vi "CylSetSeq.vi"(8 "error in (no error)":errorcluster, 9 "Delay Time":dbl[unit] format="%.3f", 10 "SEQ in":refnum<class "Sequence.lvclass">, 11 "Cycle in":refnum<class "Cycle.lvclass">) -> (0 "error out":errorcluster, 3 "Cycle out":refnum<class "Cycle.lvclass">)   [LabVIEW 2012, in "Cycle.lvclass"]
uses:
  Cycle.lvclass
  Sequence.lvclass
  Cycle.lvclass/Cycle.ctl
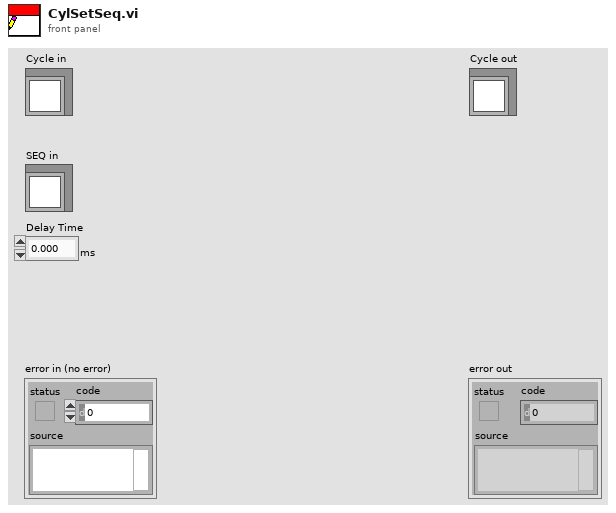
[diagram p1: front panel]
types:
  T1 = cluster{"Sequence.lvclass":refnum<class "Sequence.lvclass">, "Delay Time":dbl[unit]}[]
  T2 = cluster{"SEQ in":refnum<class "Sequence.lvclass">, "Delay Time":dbl[unit]}
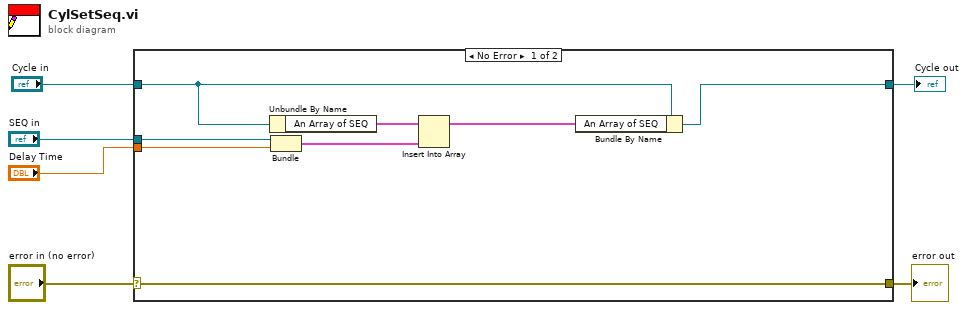
[diagram p0: block diagram]
diagram:
  n1 = case shown="No Error" "error in (no error)" {
    selector: "error in (no error)" -> [w14 w15]
    tunnel: [w14 w15] -> w5
    tunnel: [w13 w16] -> w3
    tunnel: "Cycle in" -> [w12 w16]
    tunnel: "SEQ in" -> [w9 _]
    tunnel: "Delay Time" -> [w8 _]
    frame No Error {
      n2 = Unbundle By Name(w12) -> ("An Array of SEQ"=w11:T1)
      n3 = Bundle("SEQ in"=w9, "Delay Time"=w8) -> (w10:T2)  [unwired: 1 in]
      n4 = Insert Into Array(array=w11, new element=w10) -> (w7:T1)  [unwired: 1 in]
      n5 = Bundle By Name(cluster=w12, "An Array of SEQ"=w7) -> (w13:refnum<class "Cycle.lvclass">)
    }
    frame Error {
    }
  }
  "error out" <- w5
  "Cycle out" <- w3
